vi "Text Callback.vi"(4 "User Parameter":variant, 5 "Event Data":cluster{"sender":refnum<k24>, "e":refnum<k24>}, 6 "Control Ref":refnum<k24>, 7 "Event Common Data":T1) -> ()   [LabVIEW 2018]
uses:
  System.Speech
  Data Def/Voice Control Reference.ctl
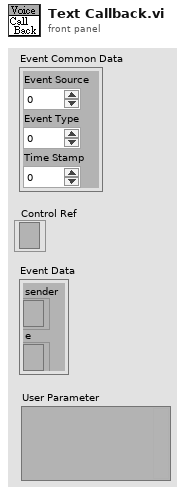
[diagram p1: front panel]
types:
  T1 = cluster{"Event Source":i32, "Event Type":u32, "Time Stamp":u32}
  T2 = typedef "Voice Control Reference.ctl" = cluster{"String in":refnum<vi>, "Score in":refnum<vi>}
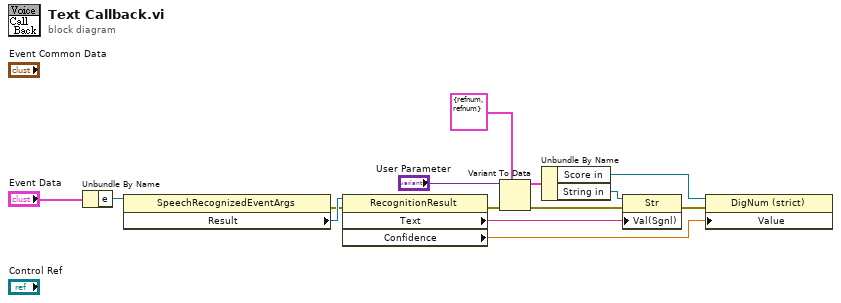
[diagram p0: block diagram]
diagram:
  n1 = Unbundle By Name("Event Data") -> ("e"=w9:refnum<k24>)
  n2 = property class="SpeechRecognizedEventArgs"(reference=w9) -> (error out=w11:errorcluster, "Result"=w12:refnum<k24>)  [unwired: 1 in, 1 out]
  n3 = property class="RecognitionResult"(reference=w12, error in=w11) -> (error out=w7:errorcluster, "Text"=w10:string, "Confidence"=w14:sgl)  [unwired: 1 out]
  n4 = Variant To Data(error in=w7, type=T2 {"String in"=refnum, "Score in"=refnum} ("Main Control Reference"), Variant="User Parameter") -> (data=w4:T2, error out=w3:errorcluster)
  n5 = Unbundle By Name(w4) -> ("Score in"=w1:refnum<vi>, "String in"=w2:refnum<vi>)
  n6 = property class="Str"(reference=w2, error in=w3, "Val(Sgnl)"=w10) -> (error out=w13:errorcluster)  [unwired: 1 out]
  n7 = property class="DigNum (strict)"(reference=w1, error in=w13, "Value"=w14) -> ()  [unwired: 2 out]
